vi "RemoveFromGroup Value Change.vi"(11 "References":T1) -> (0 "error out":errorcluster)   [LabVIEW 2015, in "TDMS datalogger editor node.lvclass"]
uses:
  TDMS datalogger editor node.lvclass
  <vilib>/NI/DCAF/Tag Editor Core/Table API/Table Manager/object ref.ctl
  <vilib>/NI/DCAF/Tag Editor Core/Configuration Editor/Classes/Engine Parent/Engine Parent Editor Node.lvclass
  <vilib>/NI/DCAF/Tag Editor Core/Configuration Editor/Classes/Module editor node/module editor node.lvclass
  TDMS datalogger editor node.lvclass/TDMS datalogger editor node.ctl
  <vilib>/NI/Tag Bus/tag/tag descriptor.lvclass/tag descriptor.ctl
  <vilib>/NI/Tag Bus/tag/tag descriptor.lvclass
  module/configuration/TDMS datalogger configuration.lvclass
  <vilib>/NI/DCAF/Tag Editor Core/Table API/Table Manager/Table Manager.lvclass
panel:
  in  "Groups":string(tree)="group1"
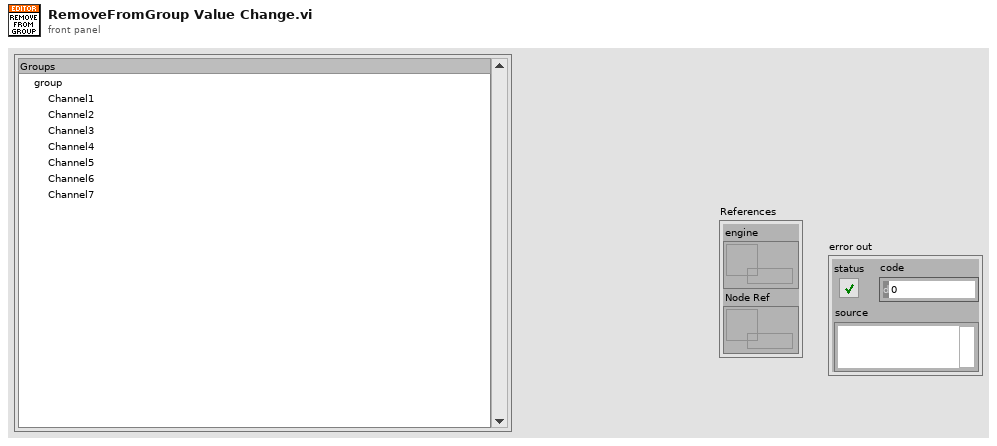
[diagram p1: front panel]
types:
  T1 = typedef "Table Manager.lvlib/Table Manager.lvclass/object ref.ctl" = cluster{"engine":refnum<data-value>, "Node Ref":refnum<data-value>}
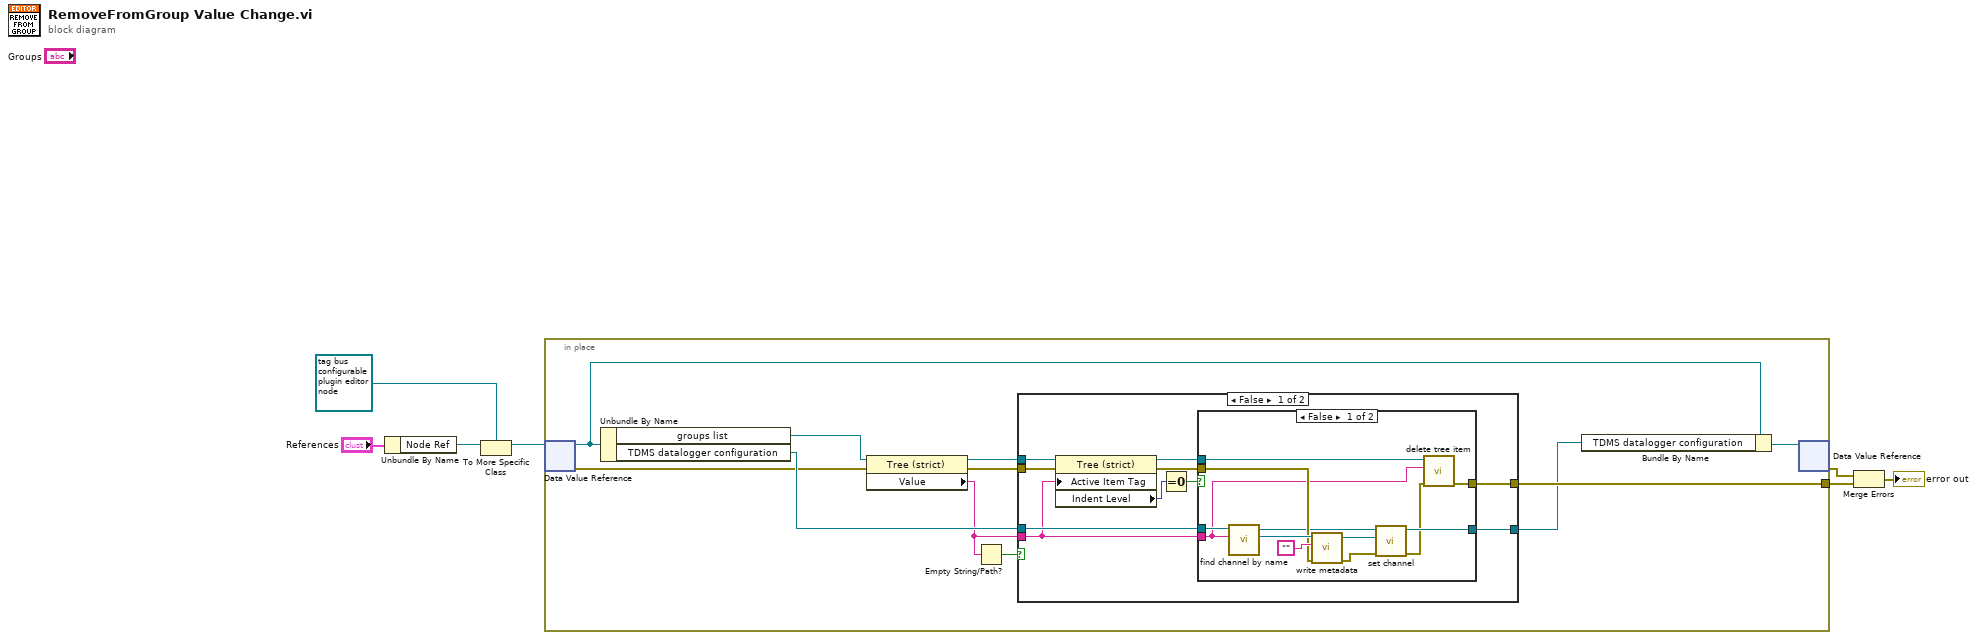
[diagram p0: block diagram]
diagram:
  n1 = Unbundle By Name("References") -> ("Node Ref"=w4:refnum<data-value>)
  n2 = To More Specific Class(target class=refnum<data-value> refnum ("data value reference"), reference=w4) -> (specific class reference=w2:refnum<data-value>)  [unwired: 1 in, 1 out]
  n3 = in-place {
    in-place-border: [w18] -> w7
    n4 = in-place-dvr #1(w2) -> (w16:refnum<class "TDMS datalogger editor node.lvclass">, w11:errorcluster)
    n5 = Unbundle By Name(w16) -> ("groups list"=w10:refnum<vi>, "TDMS datalogger configuration"=w17:refnum<class "TDMS datalogger configuration.lvclass">)
    n6 = property class="Tree (strict)"(reference=w10, error in=w11) -> (reference out=w8:refnum<vi>, error out=w12:errorcluster, "Value"=w9:string)
    n7 = Empty String/Path?(string/path=w9) -> (empty?=w13:bool)
    n8 = case shown="False" w13 {
      tunnel: [w28 w44] -> w18
      tunnel: w8 -> [w27 _]
      tunnel: w12 -> [w25 w44]
      tunnel: w17 -> [w24 w43]
      tunnel: w9 -> [w20 _]
      tunnel: [w19 w43] -> w14
      frame False {
        n9 = property class="Tree (strict)"(reference=w27, error in=w25, "Active Item Tag"=w20) -> (reference out=w26:refnum<vi>, error out=w23:errorcluster, "Indent Level"=w22:i32)
        n10 = Equal To 0?(x=w22) -> (x = 0?=w21:bool)
        n11 = case shown="False" w21 {
          tunnel: [w31 w42] -> w28
          tunnel: w26 -> [w30 _]
          tunnel: w24 -> [w40 w41]
          tunnel: w20 -> [w29 _]
          tunnel: w23 -> [w37 w42]
          tunnel: [w34 w41] -> w19
          frame False {
            n12 = call "find channel by name.vi"("channel name"=w29, "TDMS datalogger configuration in"=w40) -> ("channel"=w39:refnum<class "TBM channel.lvclass">, "TDMS datalogger configuration out"=w35:refnum<class "TDMS datalogger configuration.lvclass">)  [unwired: 8 in]
            n13 = call <vilib>:"write metadata.vi"("error in"=w37, "metadata"="", "system tag in"=w39) -> ("error out"=w33:errorcluster, "system tag out"=w36:refnum<class "TBM channel.lvclass">)  [unwired: 7 in]
            n14 = call "set channel.vi"("error in"=w33, "TBM channel in"=w36, "TDMS datalogger configuration in"=w35) -> ("error out"=w32:errorcluster, "TDMS datalogger configuration out"=w34:refnum<class "TDMS datalogger configuration.lvclass">)  [unwired: 7 in]
            n15 = call "delete tree item.vi"("error in"=w32, "Tag"=w29, "tree reference in"=w30) -> ("error out"=w31:errorcluster)  [unwired: 7 in, 1 out]
          }
          frame True {
            # "Do nothing on group items"
          }
        }
      }
      frame True {
        # "Do Nothing if no item selected"
      }
    }
    n16 = Bundle By Name(cluster=w16, "TDMS datalogger configuration"=w14) -> (w15:refnum<class "TDMS datalogger editor node.lvclass">)
    n17 = in-place-dvr #1(w15) -> (w6:errorcluster)  [unwired: 1 out]
  }
  n18 = Merge Errors(w6, w7) -> (→"error out":errorcluster)
